vi "GetPoints.vi"(1 "Input List of UTM locations to be arranged into segments":T1[](array[typedef]) {"North" format="%#_10f"; "East" format="%#_8f"}) -> (0 "Obstacle.lvclass":refnum<class "Obstacle.lvclass">)   [LabVIEW 2012, in "Obstacle.lvclass"]
doc: "Gets an input of a list of points, outputs an obstacle. Final segment is the last and first segments."
uses:
  Obstacle.lvclass
  Data/TypeDefs/UTM Location.ctl
  Obstacle.lvclass/Obstacle.ctl
panel:
  in  "Cluster 6":cluster{"Point 1":T1, "Point 0":T1} {"Point 0"."North" format="%#_10f"; "Point 0"."East" format="%#_8f"; "Point 1"."North" format="%#_10f"; "Point 1"."East" format="%#_8f"}
  in  "Obstacle.lvclass 2":refnum<class "Obstacle.lvclass">
  in  "Cluster":cluster{"Point 1":T1, "Point 0":T1} {"Point 0"."North" format="%#_10f"; "Point 0"."East" format="%#_8f"; "Point 1"."North" format="%#_10f"; "Point 1"."East" format="%#_8f"}
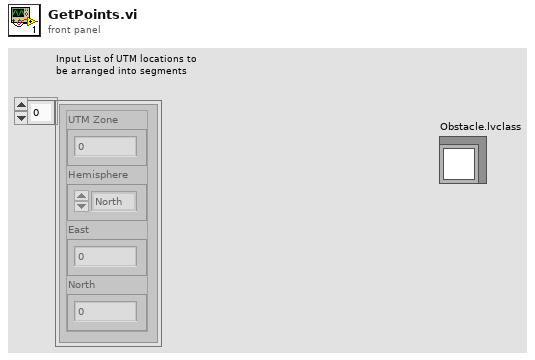
[diagram p1: front panel]
types:
  T1 = typedef "UTM Location.ctl" = cluster{"UTM Zone":dbl, "Hemisphere":enum16{"North", "South"}, "East":dbl, "North":dbl}
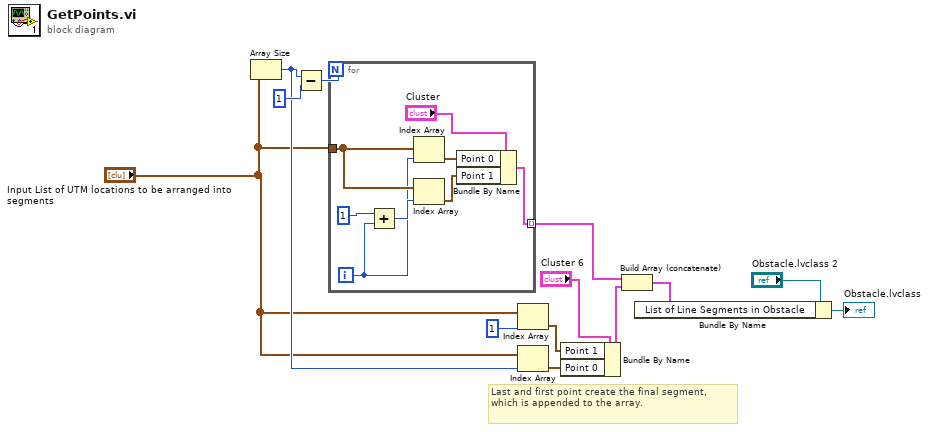
[diagram p0: block diagram]
diagram:
  # "Last and first point create the final segment, which is appended to the array."
  n1 = Array Size(array="Input List of UTM locations to be arranged into segments") -> (size(s)=w11:i32)
  n2 = Subtract(x=w11, y=1) -> (x-y=w13:i32)
  n3 = for {
    N: w13 -> [_]
    tunnel: "Input List of UTM locations to be arranged into segments" -> [w21]
    tunnel: [w15] -> w5 mode=indexing
    i -> [w18]
    n4 = Add(x=1, y=w18) -> (x+y=w20:i32)
    n5 = Index Array(array=w21, index=w18) -> (element=w17:T1)
    n6 = Index Array(array=w21, index=w20) -> (element=w16:T1)
    n7 = Bundle By Name(cluster="Cluster", "Point 0"=w17, "Point 1"=w16) -> (w15:cluster{"Point 1":T1, "Point 0":T1})
  }
  n8 = Index Array(array="Input List of UTM locations to be arranged into segments", index=1) -> (element=w7:T1)
  n9 = Index Array(array="Input List of UTM locations to be arranged into segments", index=w11) -> (element=w6:T1)
  n10 = Bundle By Name(cluster="Cluster 6", "Point 1"=w7, "Point 0"=w6) -> (w4:cluster{"Point 1":T1, "Point 0":T1})
  n11 = Build Array (concatenate)(w5, w4) -> (w3:cluster{"Point 1":T1, "Point 0":T1}[])
  n12 = Bundle By Name(cluster="Obstacle.lvclass 2", "List of Line Segments in Obstacle"=w3) -> (→"Obstacle.lvclass":refnum<class "Obstacle.lvclass">)
